vi "NPC3SG Get Positions v10.6.1.vi"(0 "Drive Visa Name":refnum<visa-resource-name>="COM5") -> (5 "Drive Current Values":T1 {"Drive Z Position" min=-273.0 max=300000.0 step=0.0001 format="%.3f"; "Drive Y Position" min=-273.0 max=300000.0 step=0.0001 format="%.3f"; "Drive X Position" min=-273.0 max=300000.0 step=0.0001 format="%.3f"})   [LabVIEW 2010]
uses:
  TypeDefs/NPC3SG Current Values.ctl
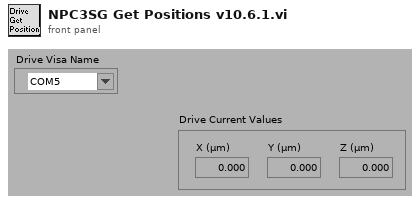
[diagram p1: front panel]
types:
  T1 = typedef "NPC3SG Current Values.ctl" = cluster{"Drive X Position":dbl, "Drive Y Position":dbl, "Drive Z Position":dbl}
  T2 = typedef "NPC3SG Current Voltages v10.6.1.ctl" = cluster{"Drive X Voltage":dbl, "Drive Y Voltage":dbl, "Drive Z Voltage":dbl}
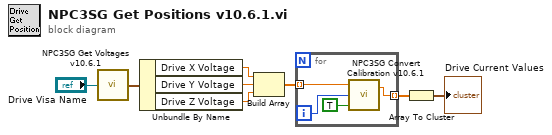
[diagram p0: block diagram]
diagram:
  n1 = call "NPC3SG Get Voltages v10.6.1.vi"("Drive Visa Name"="Drive Visa Name") -> ("Drive Current Voltages"=w2:T2)
  n2 = Unbundle By Name(w2) -> ("Drive X Voltage"=w3:dbl, "Drive Y Voltage"=w4:dbl, "Drive Z Voltage"=w5:dbl)
  n3 = Build Array(w3, w4, w5) -> (w6:dbl[])
  n4 = for {
    tunnel: w6 -> [w11] mode=indexing
    tunnel: [w10] -> w7 mode=indexing
    i -> [w9]
    n5 = call "NPC3SG Convert Calibration v10.6.1.vi"("Is Voltage?"=TRUE, "Axis"=w9, "Input Value"=w11) -> ("Output Value"=w10:dbl)  [unwired: 1 out]
  }
  n6 = Array To Cluster(array=w7) -> (cluster=→"Drive Current Values":cluster{"[0]":dbl, "[1]":dbl, "[2]":dbl})
